vi "GetGrp Devices.vi"(8 "error in (no error)":errorcluster, 10 "Selected Rows":i32[](array[numeric]), 11 "ChanGrp.lvclass":refnum<class "ChanGrp.lvclass">) -> (0 "error out":errorcluster, 3 "Dev Array":string[](array[string]))   [LabVIEW 2018, in "Configuration Grandmaster.lvlib" / "ChanGrp.lvclass"]
uses:
  ChanGrp.lvclass
  ChanGrp.lvclass/ChanGrp.ctl
  Measurements/Class Channel/Read Device.vi
  Measurements/Class Channel/Channel.lvclass
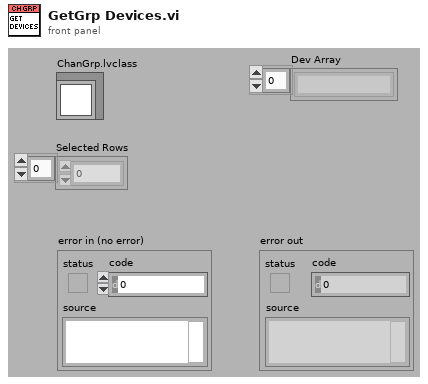
[diagram p1: front panel]
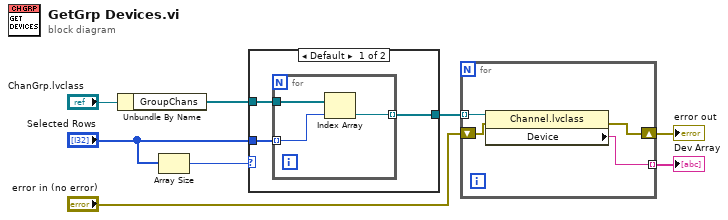
[diagram p0: block diagram]
diagram:
  n1 = Unbundle By Name("ChanGrp.lvclass") -> ("GroupChans"=w8:refnum<class "Channel.lvclass">[])
  n2 = Array Size(array="Selected Rows") -> (size(s)=w6:i32)
  n3 = case shown="Default" w6 {
    tunnel: w8 -> [w10 w15]
    tunnel: [w9 w15] -> w4
    tunnel: "Selected Rows" -> [w11 _]
    frame Default {
      n4 = for {
        tunnel: w11 -> [w13] mode=indexing
        tunnel: w10 -> [w14]
        tunnel: [w12] -> w9 mode=indexing
        n5 = Index Array(array=w14, index=w13) -> (element=w12:refnum<class "Channel.lvclass">)
      }
    }
    frame 0 {
    }
  }
  n6 = for {
    tunnel: w4 -> [w19] mode=indexing
    tunnel: [w18] -> w3 mode=indexing
    shift-right: [w16] -> w1
    shift-left: "error in (no error)" -> [w17]
    n7 = property class="Channel.lvclass"(reference=w19, error in=w17) -> (error out=w16:errorcluster, "Device"=w18:string)  [unwired: 1 out]
  }
  "Dev Array" <- w3
  "error out" <- w1
